vi "TempDAQ.vi"() -> (2 "Array":dbl[](array[numeric]))   [LabVIEW 2013]
panel:
  out "Waveform Chart":waveform(dbl)(graph)
  out "Tested Signals":dynamicdata(graph)
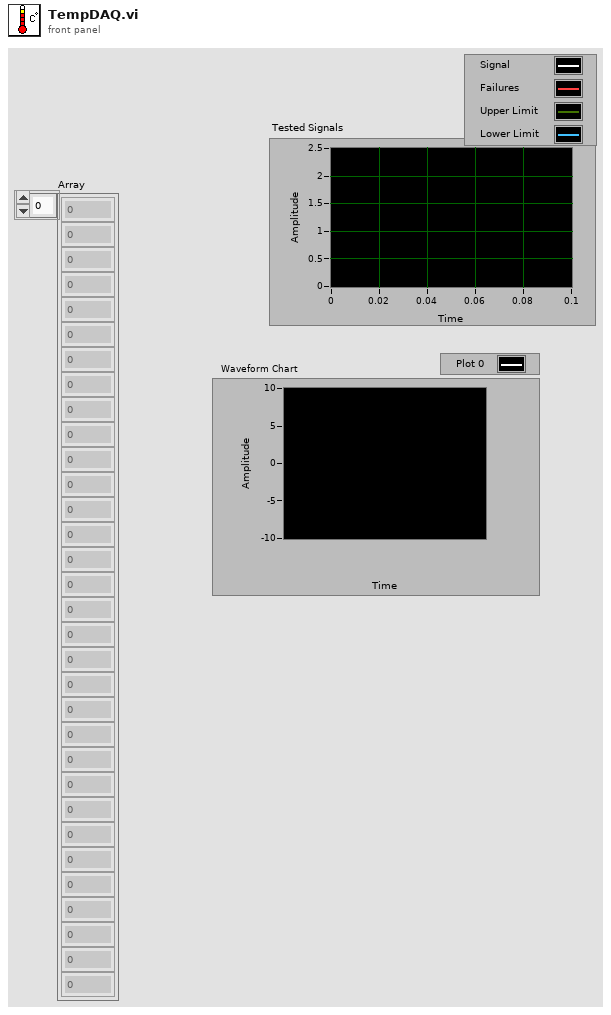
[diagram p1: front panel]
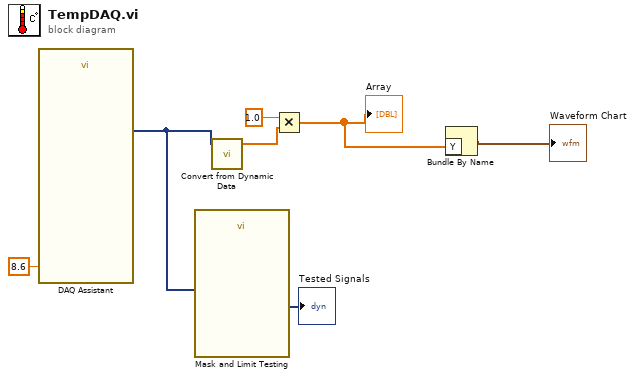
[diagram p0: block diagram]
diagram:
  n1 = call "DAQ Assistant"("timeout (s)"=8.6) -> ("data"=w4:dynamicdata)  [unwired: 16 in, 2 out]
  n2 = call "Mask and Limit Testing"("Signals"=w4) -> ("Tested Signals"=→"Tested Signals":dynamicdata)  [unwired: 7 in, 3 out]
  n3 = call "Convert from Dynamic Data"("Dynamic Data Type"=w4) -> ("Array"=w6:dbl[])  [unwired: 3 in]
  n4 = Multiply(x=1.0, y=w6) -> (x*y=w2:dbl[])
  "Array" <- w2
  n5 = Bundle By Name("Y"=w2) -> (→"Waveform Chart":waveform(dbl))  [unwired: 1 in]
